vi "Aurora Read RX0 FIFO.vi"(6 "Ready for Output (T)":bool=TRUE, 11 "Aurora FIFO":refnum<k21>) -> (0 "Output Valid":bool, 3 "Data":bool[](array[boolean]))   [LabVIEW 2019, in "FPGA Utility.lvlib"]
uses:
  <vilib>/rvi/DataTransferAndStorage/Container/Common/niFpgaContainerExecOnDevCompGetState.vi
  <vilib>/rvi/Emulation/niFpgaEmulationIsFPGAContextNoSignature.vi
  <vilib>/rvi/Emulation/niFpgaSctlEmulationGetInTimedLoop.vi
  <vilib>/rvi/errors/niFpgaSetErrorForExecOnDevCompSimple.vi
  <vilib>/rvi/eio/common/nirviEmuReportErrorAndStop.vi
  <vilib>/rvi/DataTransferAndStorage/Container/Common/niFpgaContainerGetUniqueNameForEmu.vi
  <vilib>/rvi/FIFO/Fifo_Resource/nirvififoEmulationSetSize.vi
  <vilib>/rvi/FIFO/Fifo_Resource/nirviFifoEmulationQueueMgr.vi
  <instcachedir>/0/nirviFifoEmulationQueueMgr_E5CAEC123FF24DC58D834DCA3CDAA9B5.lvgen/nirviFifoEmulationQueueMgr_E5CAEC123FF24DC58D834DCA3CDAA9B5_008.vi
  <vilib>/rvi/FIFO/Fifo_Resource/nirvififoEmulationDetermineInputValidOut.vi
  <vilib>/rvi/FIFO/Fifo_Resource/nirvififoEmulationCreateLock.vi
  <vilib>/rvi/Emulation/niFpgaProcessEmulError.vi
  <vilib>/rvi/FIFO/Fifo_Resource/nirvififoEmulationObtainLock.vi
  <vilib>/rvi/FIFO/Fifo_Resource/nirvififoEmulationReleaseLock.vi
  <vilib>/rvi/occurrence/nirviWaitOnOccurrenceBase.vi
  <vilib>/rvi/errors/nirviReportUnexpectedCaseInternalError.vi
  <vilib>/rvi/errors/nirviReportUnexpectedCaseInternalError (U32).vi
  <vilib>/Utility/error.llb/Clear Errors.vi
  <vilib>/rvi/interface/RandomDataEmulation/niFpgaRandomDataHandleErrors.vi
  <vilib>/rvi/DataTransferAndStorage/Container/XNode/niFpgaContainer.xnode
  <vilib>/rvi/FIFO/Fifo_Resource/niFpgaFifoEmulationRefIn.vi
  FPGA Utility.lvlib
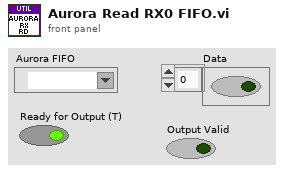
[diagram p1: front panel]
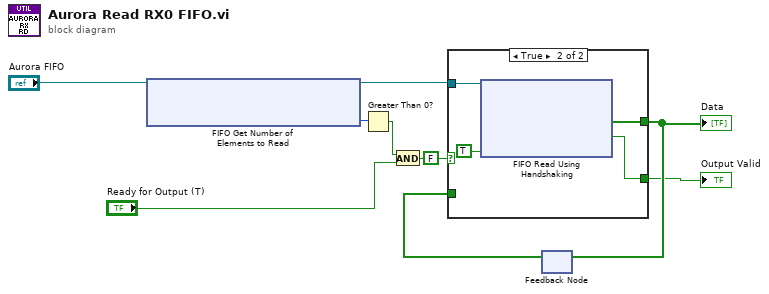
[diagram p0: block diagram]
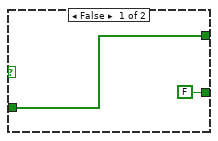
[diagram p2: hidden frame]
diagram:
  (unwired) FALSE
  n1 = xnode "FIFO Get Number of Elements to Read"("FIFO In"="Aurora FIFO") -> ("Number of Elements to Read"=w1:u32, "FIFO Out"=w6:refnum<k21>)
  n2 = Greater Than 0?(x=w1) -> (x > 0?=w7:bool)
  n3 = And(x=w7, y="Ready for Output (T)") -> (x .and. y?=w8:bool)
  n4 = feedback #1() -> (w4:bool[])  [unwired: 1 in]
  n5 = case shown="True" w8 {
    tunnel: [FALSE ("Output Valid") w14] -> w2
    tunnel: w4 -> [w11 _]
    tunnel: [w11 w13] -> w3
    tunnel: w6 -> [_ w12]
    frame False {
    }
    frame True {
      n6 = xnode "FIFO Read Using Handshaking"("Ready for Output"=TRUE, "FIFO In"=w12) -> ("Element"=w13:bool[], "Output Valid"=w14:bool)  [unwired: 1 out]
    }
  }
  "Data" <- w3
  "Output Valid" <- w2
  n7 = feedback-in #1(w3) -> ()
